vi "GenerateMessageBody.vi"(8 "error in (no error)":errorcluster, 10 "Message":T1, 11 "VI reference":refnum<vi>) -> (0 "error out":errorcluster)   [LabVIEW 2017, in "MessageGen.lvlib"]
uses:
  <vilib>/addons/InsightCM/MessageBus/CodeGen/MessageGen.lvlib
  <vilib>/addons/InsightCM/MessageBus/CodeGen/controls/MessageData.ctl
  <vilib>/addons/InsightCM/MessageBus/CodeGen/controls/MessageType.ctl
  <vilib>/addons/InsightCM/MessageBus/CodeGen/controls/Parameter.ctl
  <vilib>/addons/InsightCM/MessageBus/CodeGen/controls/ParameterType.ctl
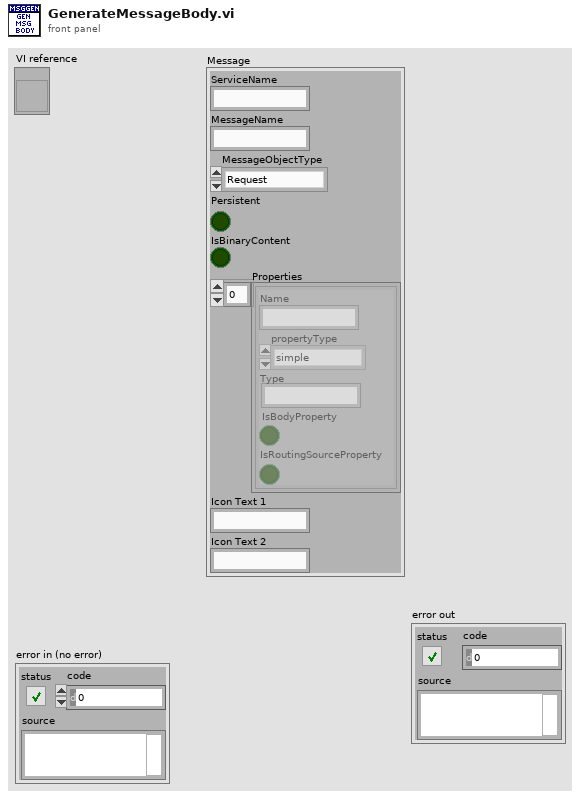
[diagram p1: front panel]
types:
  T1 = typedef "MessageGen.lvlib/MessageData.ctl" = cluster{"ServiceName":string, "MessageName":string, "MessageObjectType":T2, "Persistent":bool, "IsBinaryContent":bool, "Properties":T3[], "Icon Text 1":string, "Icon Text 2":string}
  T2 = typedef "MessageGen.lvlib/MessageType.ctl" = enum16{"Request", "Response", "Broadcast", "RoutedMessage"}
  T3 = typedef "MessageGen.lvlib/Parameter.ctl" = cluster{"Name":string, "propertyType":T4, "Type":string, "IsBodyProperty":bool, "IsRoutingSourceProperty":bool}
  T4 = typedef "MessageGen.lvlib/ParameterType.ctl" = enum16{"simple", "bytearray", "dateTime", "list", "map", "object"}
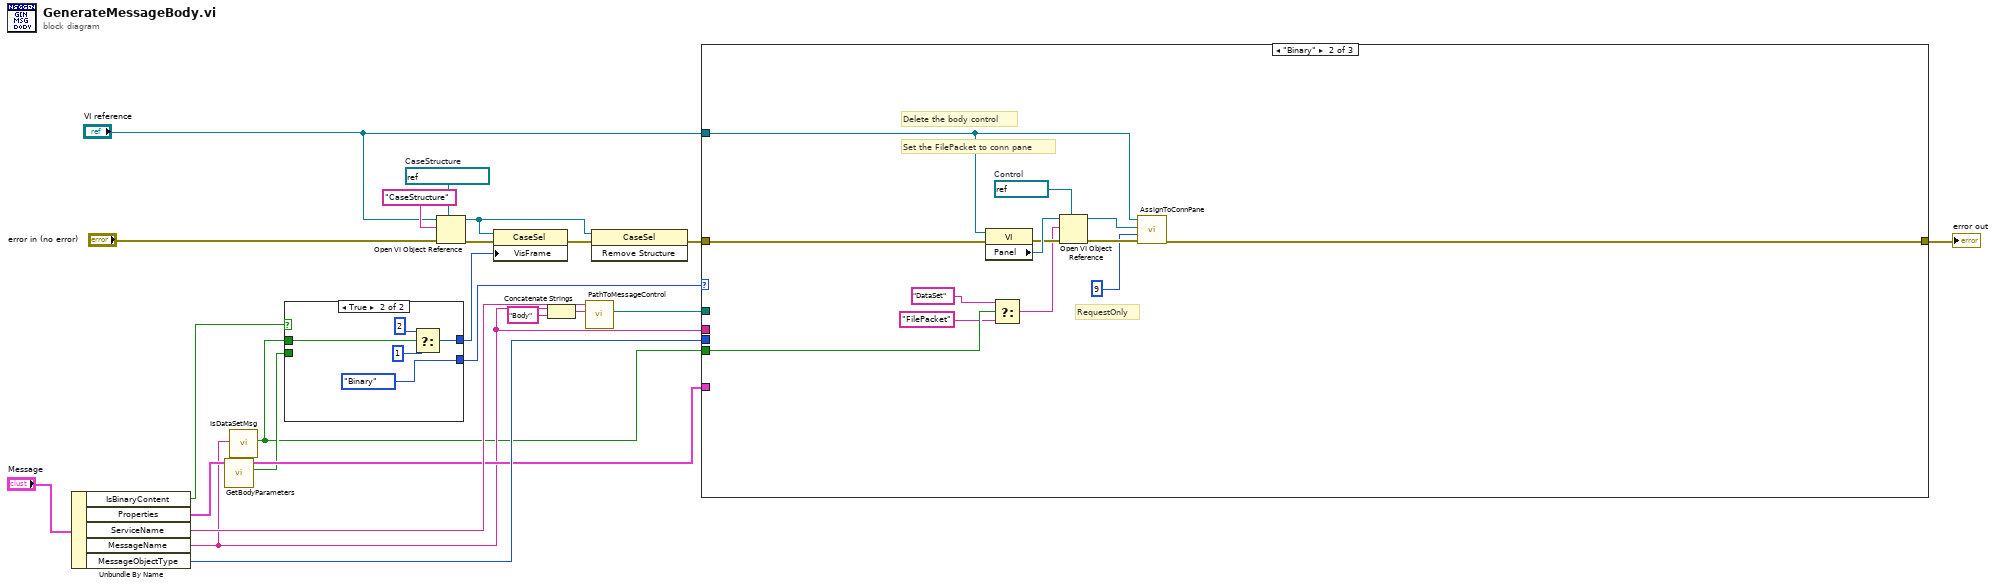
[diagram p0: block diagram]
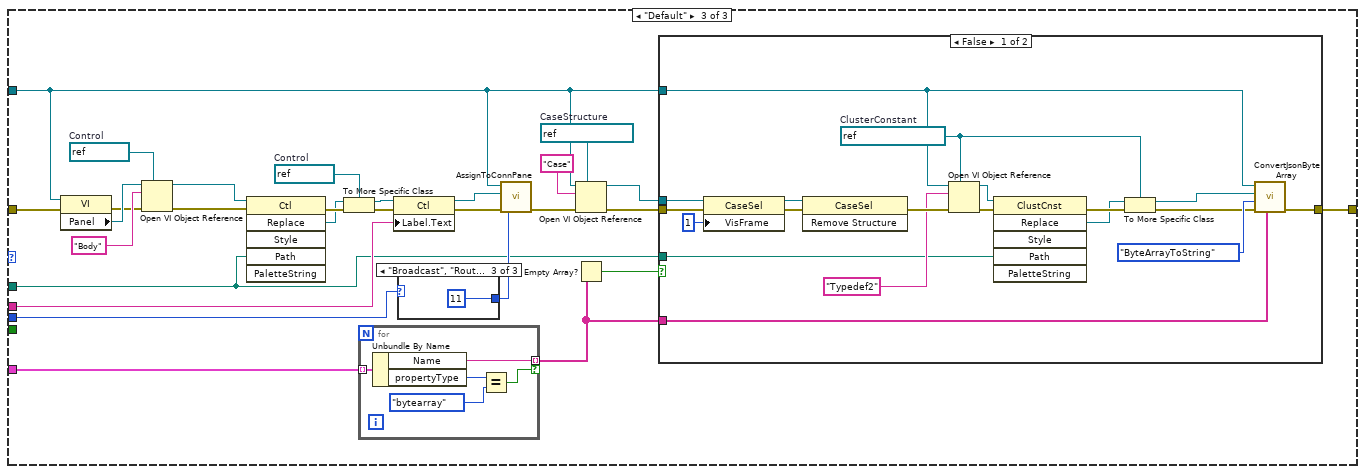
[diagram p3: hidden frame]
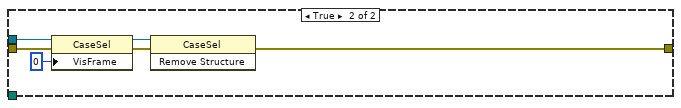
[diagram p4: hidden frame]
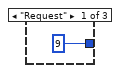
[diagram p5: hidden frame]
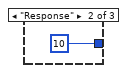
[diagram p6: hidden frame]
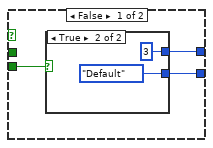
[diagram p7: hidden frame]
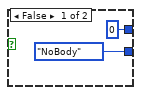
[diagram p8: hidden frame]
diagram:
  w18 = refnum<vi> refnum  # CaseStructure
  n1 = Unbundle By Name("Message") -> ("IsBinaryContent"=w6:bool, "Properties"=w17:T3[], "ServiceName"=w13:string, "MessageName"=w2:string, "MessageObjectType"=w10:T2)
  n2 = call <vilib>:"GetBodyParameters.vi"("Parameters"=w17) -> ("HasBodyParameters"=w5:bool, "BodyParameters"=w9:T3[])  [unwired: 9 in]
  n3 = call <vilib>:"IsDataSetMsg.vi"("MessageName"=w2) -> ("IsDataSet"=w1:bool)  [unwired: 10 in]
  n4 = case shown="True" w6 {
    tunnel: w5 -> [w26 _]
    tunnel: [w25 enum16{"NoBody", "Binary", "Default"}."Binary"] -> w16
    tunnel: [w24 w32] -> w3
    tunnel: w1 -> [_ w31]
    frame False {
      n5 = case shown="True" w26 {
        tunnel: [enum16{"NoBody", "Binary", "Default"}."NoBody" enum16{"NoBody", "Binary", "Default"}."Default"] -> w25
        tunnel: [u32 0 ("Visible Frame") u32 3 ("Visible Frame")] -> w24
        frame False {
        }
        frame True {
        }
      }
    }
    frame True {
      n6 = Select(t=u32 2 ("Visible Frame"), s=w31, f=u32 1 ("Visible Frame")) -> (s? t:f=w32:u32)
    }
  }
  n7 = Open VI Object Reference(7:w18, 8:"error in (no error)", 10:"CaseStructure" ("name/order"), 11:"VI reference") -> (0:w22:errorcluster, 3:w21:refnum<vi>)
  n8 = property class="CaseSel"(reference=w21, error in=w22, "VisFrame"=w3) -> (error out=w20:errorcluster)  [unwired: 1 out]
  n9 = Concatenate Strings(w2, "Body" ("string")) -> (w14:string)
  n10 = call <vilib>:"PathToMessageControl.vi"("ControlName"=w14, "Service"=w13) -> ("Path"=w12:path)  [unwired: 9 in]
  n11 = invoke class="CaseSel" method="Remove Structure"(reference=w21, error in=w20) -> (error out=w11:errorcluster)  [unwired: 1 in, 2 out]
  n12 = case shown="\"Binary\"" w16 {
    tunnel: w12 -> [_ _ w59]
    tunnel: w2 -> [_ _ w70]
    tunnel: w11 -> [w36 w41 w53]
    tunnel: w10 -> [_ _ w69]
    tunnel: "VI reference" -> [_ w46 w50]
    tunnel: w9 -> [_ _ w64]
    tunnel: [w36 w42 w58] -> w8
    tunnel: w1 -> [_ w40 _]
    frame "NoBody" {
      # "Delete the body control"
    }
    frame "Binary" {
      w49 = refnum<vi> refnum  # Control
      # "RequestOnly"
      # "Set the FilePacket to conn pane"
      # "Delete the body control"
      n13 = property class="VI"(reference=w46, error in=w41) -> (error out=w47:errorcluster, "Panel"=w48:refnum<vi>)  [unwired: 1 out]
      n14 = Select(t="DataSet" ("string"), s=w40, f="FilePacket" ("string")) -> (s? t:f=w38:string)
      n15 = Open VI Object Reference(7:w49, 8:w47, 10:w38, 11:w48) -> (0:w44:errorcluster, 3:w45:refnum<vi>)
      n16 = call <vilib>:"AssignToConnPane.vi"("error in (no error)"=w44, "term index"=u32 9, "Control"=w45, "vi reference"=w46) -> ("error out"=w42:errorcluster)  [unwired: 7 in]
    }
    frame "Default" {
      w57 = refnum<vi> refnum  # Control
      w66 = refnum<vi> refnum  # CaseStructure
      w75 = refnum<vi> refnum  # Control
      n17 = property class="VI"(reference=w50, error in=w53) -> (error out=w54:errorcluster, "Panel"=w56:refnum<vi>)  [unwired: 1 out]
      n18 = Open VI Object Reference(7:w57, 8:w54, 10:"Body" ("string"), 11:w56) -> (0:w52:errorcluster, 3:w51:refnum<vi>)
      n19 = invoke class="Ctl" method="Replace"(reference=w51, error in=w52, "Path"=w59) -> (error out=w77:errorcluster, "Replace"=w76:refnum<vi>)  [unwired: 3 in, 4 out]
      n20 = To More Specific Class(target class=w75, reference=w76, error in=w77) -> (specific class reference=w72:refnum<vi>, error out=w74:errorcluster)
      n21 = for {
        tunnel: w64 -> [w107] mode=indexing
        tunnel: [w105] -> w62 mode=indexing if=w103
        n22 = Unbundle By Name(w107) -> ("Name"=w105:string, "propertyType"=w106:T4)
        n23 = Equal?(x=w106, y=ParameterType."bytearray" ("x")) -> (x = y?=w103:bool)
      }
      n24 = property class="Ctl"(reference=w72, error in=w74, "Label.Text"=w70) -> (reference out=w71:refnum<vi>, error out=w73:errorcluster)
      n25 = case shown="\"Broadcast\", \"RoutedMessage\"" w69 {
        tunnel: [u32 9 ("term index") u32 10 ("term index") u32 11 ("term index")] -> w68
        frame "Request" {
        }
        frame "Response" {
        }
        frame "Broadcast", "RoutedMessage" {
        }
      }
      n26 = call <vilib>:"AssignToConnPane.vi"("error in (no error)"=w73, "term index"=w68, "Control"=w71, "vi reference"=w50) -> ("error out"=w65:errorcluster)  [unwired: 7 in]
      n27 = Open VI Object Reference(7:w66, 8:w65, 10:"Case" ("name/order"), 11:w50) -> (0:w63:errorcluster, 3:w60:refnum<vi>)
      n28 = Empty Array?(array=w62) -> (empty?=w61:bool)
      n29 = case shown="False" w61 {
        tunnel: [w79 w97] -> w58
        tunnel: w50 -> [w88 _]
        tunnel: w63 -> [w90 w99]
        tunnel: w60 -> [w89 w98]
        tunnel: w62 -> [w86 _]
        tunnel: w59 -> [w78 _]
        frame False {
          w82 = refnum<vi> refnum  # ClusterConstant
          n30 = property class="CaseSel"(reference=w89, error in=w90, "VisFrame"=u32 1 ("Visible Frame")) -> (reference out=w92:refnum<vi>, error out=w93:errorcluster)
          n31 = invoke class="CaseSel" method="Remove Structure"(reference=w92, error in=w93) -> (error out=w94:errorcluster)  [unwired: 1 in, 2 out]
          n32 = Open VI Object Reference(7:w82, 8:w94, 10:"Typedef2" ("name/order"), 11:w88) -> (0:w96:errorcluster, 3:w95:refnum<vi>)
          n33 = invoke class="ClustCnst" method="Replace"(reference=w95, error in=w96, "Path"=w78) -> (error out=w84:errorcluster, "Replace"=w81:refnum<vi>)  [unwired: 3 in, 4 out]
          n34 = To More Specific Class(target class=w82, reference=w81, error in=w84) -> (specific class reference=w80:refnum<vi>, error out=w83:errorcluster)
          n35 = call <vilib>:"ConvertJsonByteArray.vi"("controls to convert"=w86, "error in (no error)"=w83, "direction"=enum16{"ByteArrayToString", "StringToByteArray"}."ByteArrayToString", "cluster to disconnect"=w80, "VI ref"=w88) -> ("error out"=w79:errorcluster)  [unwired: 6 in]
        }
        frame True {
          n36 = property class="CaseSel"(reference=w98, error in=w99, "VisFrame"=u32 0 ("Visible Frame")) -> (reference out=w101:refnum<vi>, error out=w102:errorcluster)
          n37 = invoke class="CaseSel" method="Remove Structure"(reference=w101, error in=w102) -> (error out=w97:errorcluster)  [unwired: 1 in, 2 out]
        }
      }
    }
  }
  "error out" <- w8
